vi "MSScript update_menu.vi"(7 "user_defined":string[](array[string]), 8 "error in (no error)":errorcluster, 11 "MenuRef":refnum<k9>) -> (0 "error out":errorcluster)   [LabVIEW 2018]
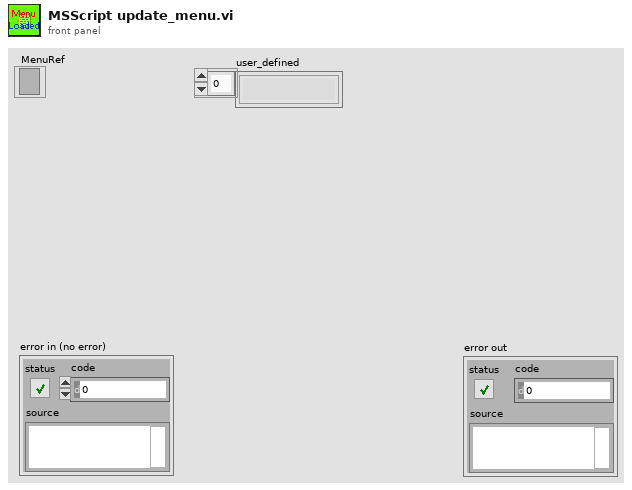
[diagram p1: front panel]
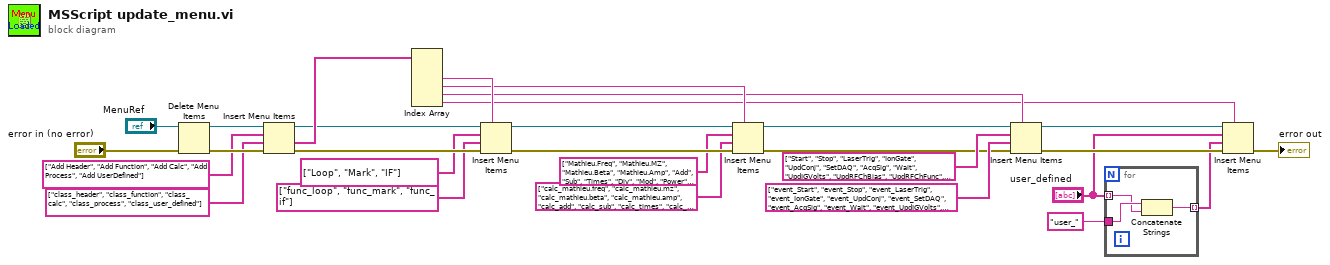
[diagram p0: block diagram]
diagram:
  n1 = Delete Menu Items(6:"error in (no error)", 9:"MenuRef") -> (0:w27:errorcluster, 3:w26:refnum<k9>)  [unwired: 2 in]
  n2 = Insert Menu Items(6:w27, 7:string[] ["class_header", "class_function", "class_calc", "class_process", "class_user_defined"] ("item tags"), 8:string[] ["Add Header", "Add Function", "Add Calc", "Add Process", "Add UserDefined"] ("item names"), 9:w26) -> (0:w20:errorcluster, 1:w23:string[], 3:w22:refnum<k9>)  [unwired: 2 in]
  n3 = Index Array(array=w23) -> (element #2=w21:string, element #3=w17:string, element #4=w12:string, element #5=w4:string)  [unwired: 5 in, 1 out]
  n4 = Insert Menu Items(5:w21, 6:w20, 7:string[] ["func_loop", "func_mark", "func_if"] ("item tags"), 8:string[] ["Loop", "Mark", "IF"] ("item names"), 9:w22) -> (0:w15:errorcluster, 3:w16:refnum<k9>)  [unwired: 1 in, 1 out]
  n5 = Insert Menu Items(5:w17, 6:w15, 7:string[] ["calc_mathieu.freq", "calc_mathieu.mz", "calc_mathieu.beta", "calc_mathieu.amp", "calc_add", "calc_sub", "calc_times", "calc_div", "calc_mod", "calc_pow", "calc_floor", "calc_ceil", "calc_max", "calc_min", "calc_sign", "calc_abs"] ("item tags"), 8:string[] ["Mathieu.Freq", "Mathieu.MZ", "Mathieu.Beta", "Mathieu.Amp", "Add", "Sub", "Times", "Div", "Mod", "Power", "Floor", "Ceil", "Max", "Min", "Sign", "Abs"] ("item names"), 9:w16) -> (0:w8:errorcluster, 3:w9:refnum<k9>)  [unwired: 1 in, 1 out]
  n6 = Insert Menu Items(5:w12, 6:w8, 7:string[] ["event_Start", "event_Stop", "event_LaserTrig", "event_IonGate", "event_UpdConj", "event_SetDAQ", "event_AcqSig", "event_Wait", "event_UpdIGVolts", "event_UpdRFChBias", "event_UpdRFChFunc", "event_UpdRFChScale", "event_UpdAuxArbPulses", "event_AuxScan", "event_PhaseScan", "event_PhaseScanII", "event_AmpScan", "event_CLFreqScan", "event_ResetRFPhase", "event_UpdAO", "event_UpdDO", "event_FGen"] ("item tags"), 8:string[] ["Start", "Stop", "LaserTrig", "IonGate", "UpdConj", "SetDAQ", "AcqSig", "Wait", "UpdIGVolts", "UpdRFChBias", "UpdRFChFunc", "UpdRFChScale", "UpdAuxArbPulses", "AuxScan", "PhaseScan", "PhaseScanII", "AmpScan", "CLFreqScan", "ResetRFPhase", "UpdAO", "UpdDO", "FGen"] ("item names"), 9:w9) -> (0:w5:errorcluster, 3:w6:refnum<k9>)  [unwired: 1 in, 1 out]
  n7 = for {
    tunnel: "user_defined" -> [w31] mode=indexing
    tunnel: "user_" ("string") -> [w32]
    tunnel: [w30] -> w2 mode=indexing
    n8 = Concatenate Strings(w32, w31) -> (w30:string)
  }
  n9 = Insert Menu Items(5:w4, 6:w5, 7:w2, 8:"user_defined", 9:w6) -> (0:→"error out":errorcluster)  [unwired: 1 in, 2 out]
